vi "FGEN-SCOPE.vi"(0 "Device Name":tag="Dev1", 1 "Amplitude":dbl caption="FGEN_Amplitude", 2 "DC Offset":dbl caption="FGEN_DC_Offset", 3 "Frequency":dbl caption="FGEN_Frequency", 4 "Waveform Type":enum16{"Sine", "Triangular", "Square"}(ring) caption="FGEN_Waveform_Type", 5 "Sample Rate (Hz)":dbl=100000.0 caption="SCOPEH_SampleRate" min=0.0 step=1000000.0 format="%#_4p", 6 "Record Length":i32=2000 caption="SCOPEH_RecordLength" min=5 max=75000000 step=1 format="%#.9p", 7 "Acquire":u16(ring)=10178 caption="SCOPEH_Acquire" items=["N Samples"=10178, "Continuously"=10123], 8 "ChA_Source":u16(ring) items=["CH0", "CH1", "CH2", "CH3"], 9 "ChB_Source":u16(ring) items=["CH4", "CH5", "CH6", "CH7"], 10 "ChA Coupling":u16(ring) caption="ChA_Coupling" items=["DC", "AC"], 11 "ChB_ Coupling":u16(ring) caption="ChB_Coupling" items=["DC", "AC"], 12 "ChA Range":dbl caption="ChA_Range", 13 "ChB Range":dbl caption="ChB_Range", 14 "ChA Offset":dbl caption="ChA_Offset", 15 "ChB Offset":dbl caption="ChB_Offset", 16 "Trigger Source":u16(ring) caption="SCOPET_Source" items=["Immediate", "TRIGGER", "SYNC_OUT", "CH A", "CH B"], 17 "Trigger Type":u16(ring) caption="SCOPET_Type" items=["Digital", "Analog"], 18 "Slope":i32(ring) caption="SCOPET_Slope" items=["Positive", "Negative"], 19 "Level":dbl caption="SCOPET_Level", 25 "SetupID":u8, 27 "input_FG_Connection":u8) -> (20 "Complete?":bool=TRUE, 24 "interleaved array":dbl[](array[numeric]))   [LabVIEW 2011]
uses:
  <vilib>/Analysis/Matrix/Datatypes/RealMatrix.ctl
  <vilib>/DAQmx/write.llb/DAQmx Write (Digital 1D Bool 1Chan 1Samp).vi
  <vilib>/DAQmx/create/channels.llb/DAQmx Create Channel (DO-Digital Output).vi
  <vilib>/DAQmx/miscellaneous.llb/DAQmx Fill In Error Info.vi
  <vilib>/Analysis/Matrix/NI_Matrix.lvlib
panel:
  out "time vector":dbl[](array[numeric])
  out "task out func":refnum<k21>
  out "CH A":T1
  out "CH B":T1
  out "Record count":i32
  out "overall scan time (seconds)":dbl
  out "Waveform Graph":dbl[][](graph)
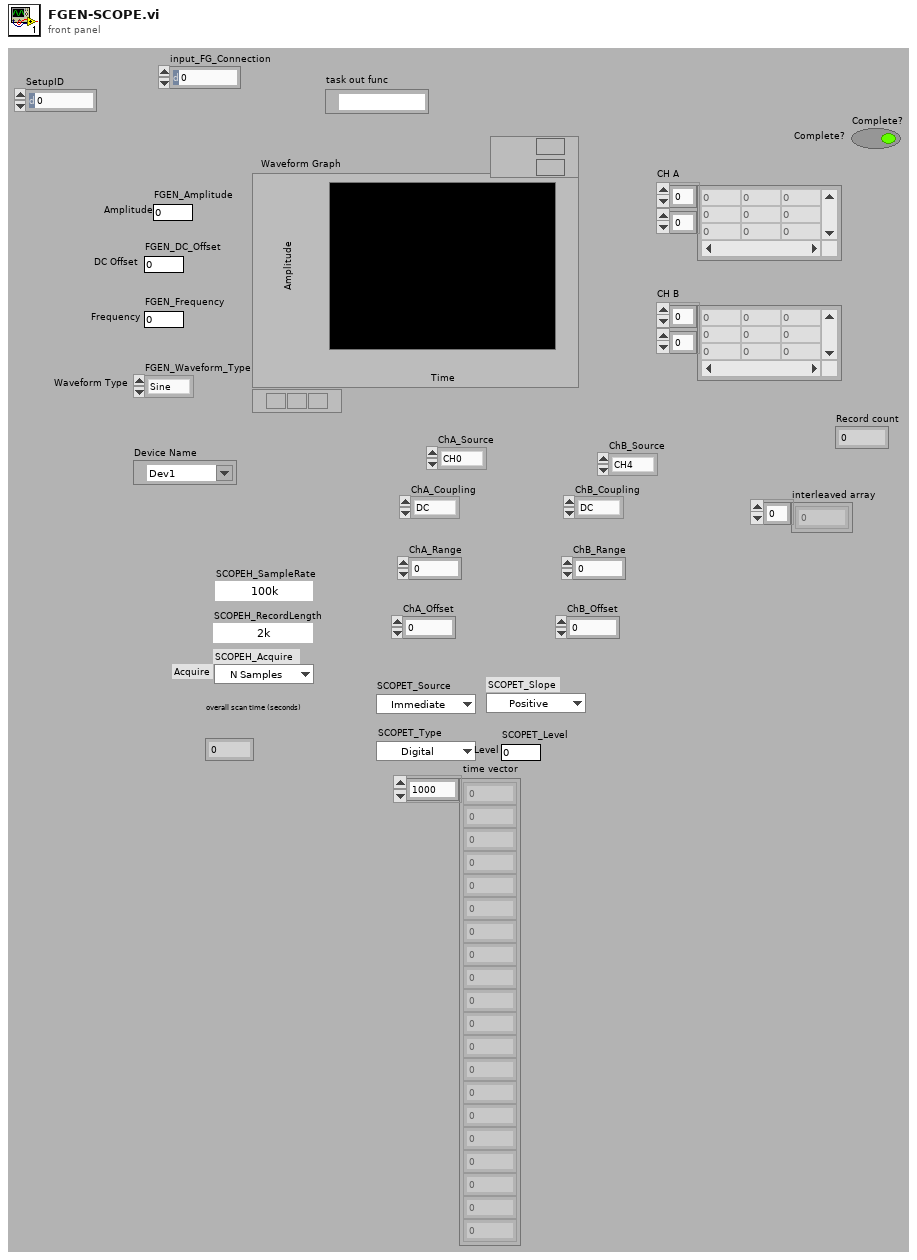
[diagram p1: front panel]
types:
  T1 = typedef "NI_Matrix.lvlib/RealMatrix.ctl" = dbl[][]
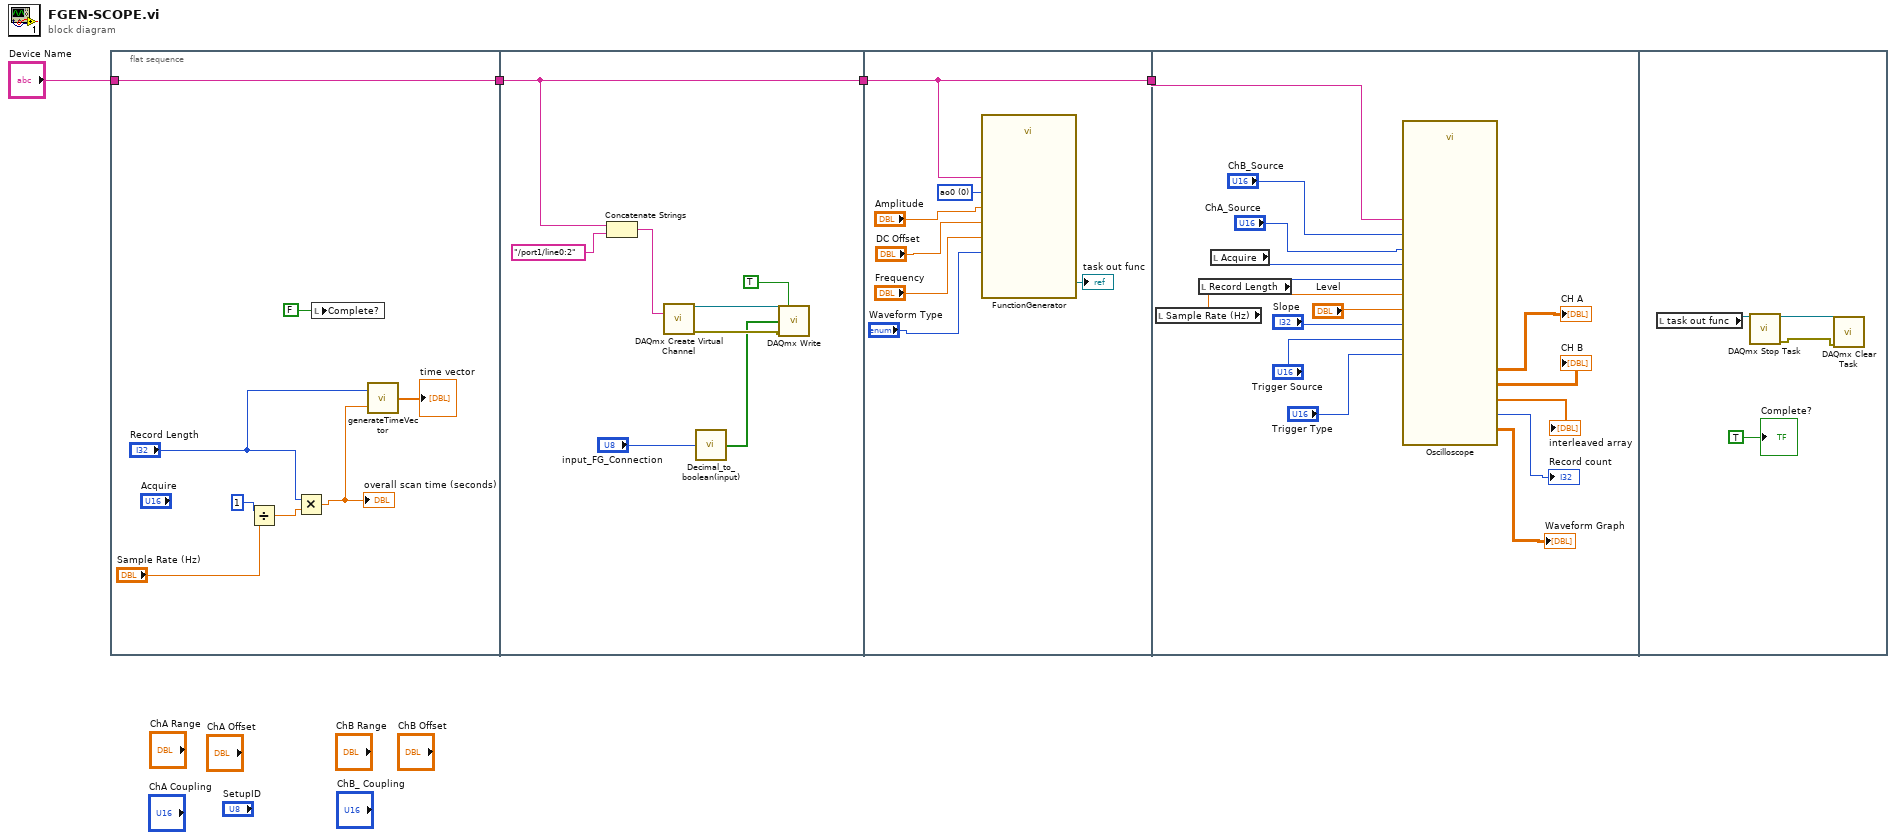
[diagram p0: block diagram]
diagram:
  n1 = flat-sequence {
    tunnel: "Device Name" -> [w12]
    tunnel: [w12] -> w1
    tunnel: [w15] -> w4
    tunnel: w1 -> [w15]
    tunnel: w4 -> [w26]
    tunnel: [w26] -> w2
    tunnel: w2 -> [w42]
    frame #0 {
      n2 = Divide(x=1, y="Sample Rate (Hz)") -> (x/y=w8:dbl)
      n3 = Multiply(x="Record Length", y=w8) -> (x*y=w6:dbl)
      "overall scan time (seconds)" <- w6
      n4 = local write "Complete?"(FALSE ("Complete?")) -> ()
      n5 = call "generateTimeVector.vi"("sampling time"=w6, "record length"="Record Length") -> ("time vector"=→"time vector":dbl[])  [unwired: 1 in]
    }
    frame #1 {
      n6 = Concatenate Strings(w15, "/port1/line0:2") -> (w14:string)
      n7 = call-poly <vilib>:"DAQmx Create Virtual Channel.vi"("lines"=w14) -> ("task out"=w20:refnum<k21>, "error out"=w19:errorcluster)  [unwired: 13 in]
      n8 = call "Decimal_to_boolean(input).vi"("conInput"="input_FG_Connection") -> ("dig IO"=w18:bool[])
      n9 = call-poly <vilib>:"DAQmx Write.vi"("task/channels in"=w20, "auto start"=TRUE, "data"=w18, "error in"=w19) -> ()  [unwired: 9 in, 3 out]
    }
    frame #2 {
      w24 = u16 0 items=["ao0", "ao1"] ("Channel")
      n10 = call "FunctionGenerator.vi"("Frequency"="Frequency", "Waveform Type"="Waveform Type", "DC Offset"="DC Offset", "Amplitude"="Amplitude", "Channel"=w24, "Device Name"=w26) -> ("task out"=→"task out func":refnum<k21>)  [unwired: 4 in, 1 out]
    }
    frame #3 {
      n11 = local read "Sample Rate (Hz)"() -> (w30:dbl)
      n12 = local read "Record Length"() -> (w32:i32)
      n13 = local read "Acquire"() -> (w31:u16)
      n14 = call "Oscilloscope.vi"("Trigger Source"="Trigger Source", "ChA_Source"="ChA_Source", "ChB_Source"="ChB_Source", "Device Name"=w42, "Trigger Type"="Trigger Type", "Slope"="Slope", "Level"="Level", "Sample Rate (Hz)"=w30, "Record Length"=w32, "Acquire"=w31) -> ("CH A"=→"CH A":T1, "CH B"=→"CH B":T1, "Record count"=→"Record count":i32, "Waveform Graph"=→"Waveform Graph":dbl[][], "interleaved array"=→"interleaved array":dbl[])  [unwired: 1 in]
    }
    frame #4 {
      n15 = local read "task out func"() -> (w44:refnum<k21>)
      n16 = call <vilib>:"DAQmx Stop Task.vi"("task/channels in"=w44) -> ("task out"=w46:refnum<k21>, "error out"=w45:errorcluster)  [unwired: 13 in]
      n17 = call <vilib>:"DAQmx Clear Task.vi"("task in"=w46, "error in"=w45) -> ()  [unwired: 13 in, 1 out]
      "Complete?" <- TRUE ("Complete?")
    }
  }
